vi "_OP_40.vi"(9 "OP_40_Integer":u16[][](array[numeric])=[[0, 0], [0, 0], [0, 0], [0, 0], [0, 0], [0, 0], [0, 0], [0, 0], [0, 0], [0, 0], [0, 0], [0, 0], [0, 0], [0, 0], [0, 0], [52429, 16268], [52429, 16268], [0, 0], [0, 0], [0, 0], [0, 0], [0, 0], [0, 0], [0, 0], [0, 0], [0, 0], [0, 0]], 10 "OP_40_Float":sgl[][](array[numeric])=[[0.0], [0.0], [0.0], [0.0], [1.38], [88.84], [0.0], [11.91], [16.25], [0.0], [0.0], [0.0], [0.0], [-30.7], [30.7], [0.0], [0.0], [-21.4], [26.7], [4.4], [21.91], [6.25], [0.0], [0.0], [0.0], [0.0], [0.0]], 11 "OP_40_string":string[](array[string])) -> (0 "Cluster":T1, 1 "Cluster 2":T1, 2 "Cluster 3":T1, 3 "Cluster 4":T1)   [LabVIEW 2024]
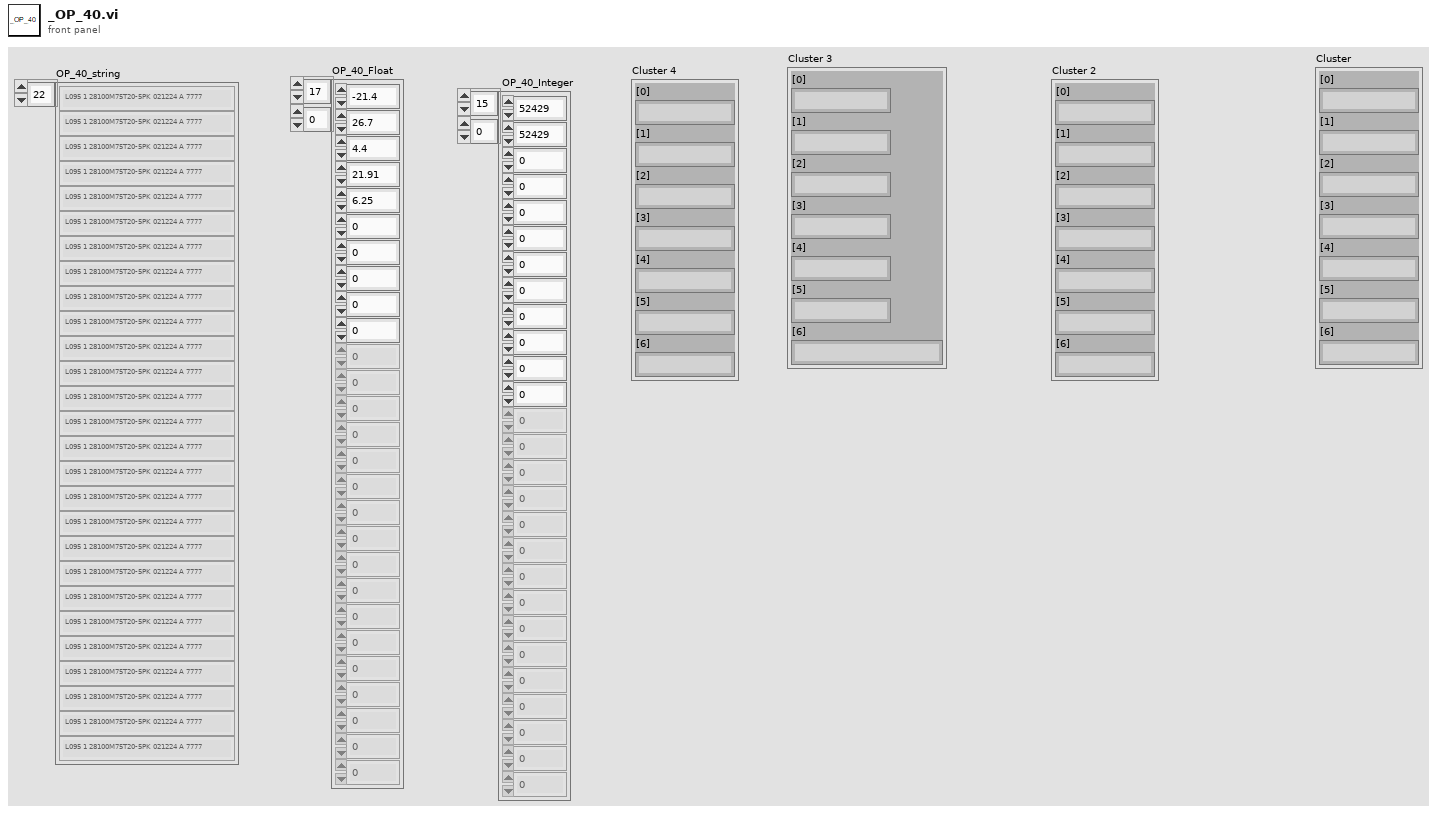
[diagram p1: front panel]
types:
  T1 = cluster{"[0]":string, "[1]":string, "[2]":string, "[3]":string, "[4]":string, "[5]":string, "[6]":string}
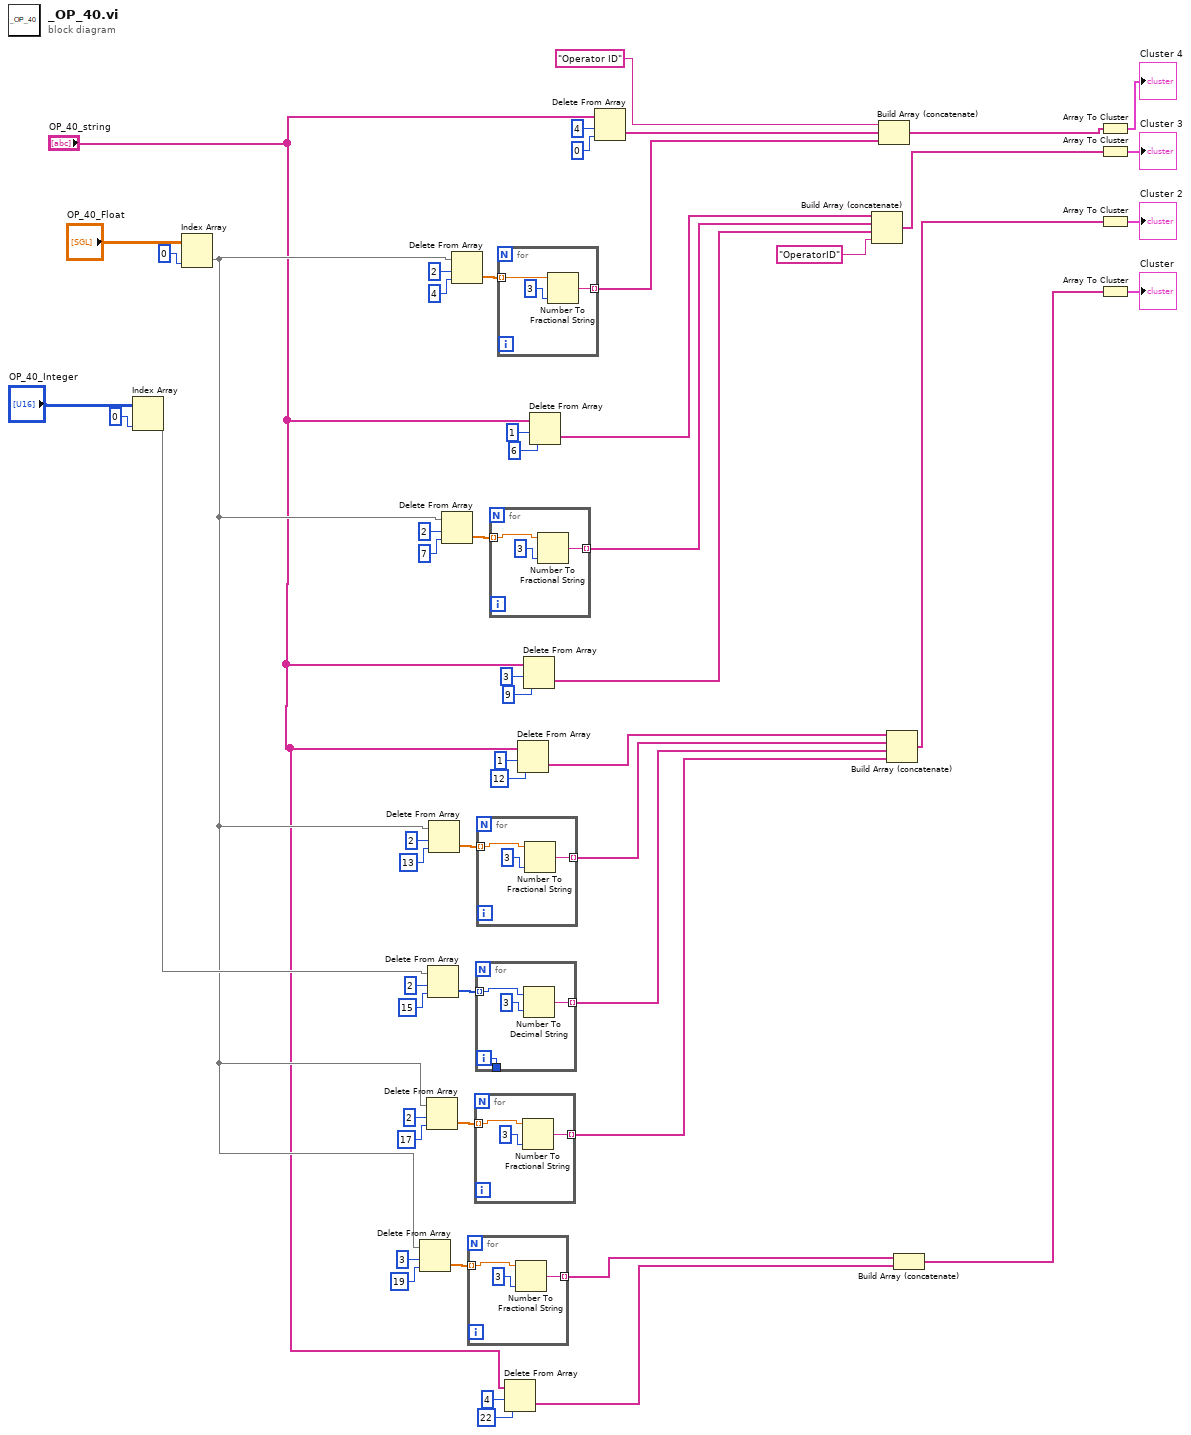
[diagram p0: block diagram]
diagram:
  n1 = Index Array(array="OP_40_Integer", index (col)=0 ("disabled index (col)")) -> (element=w17:u16[])  [unwired: 1 in]
  n2 = Index Array(array="OP_40_Float", index (col)=0 ("disabled index (col)")) -> (element=w7:sgl[])  [unwired: 1 in]
  n3 = Delete From Array(array=w7, length=3, index=19) -> (deleted portion=w10:sgl[])  [unwired: 1 out]
  n4 = Delete From Array(array=w7, length=2, index=17) -> (deleted portion=w13:sgl[])  [unwired: 1 out]
  n5 = Delete From Array(array=w17, length=2, index=15) -> (deleted portion=w20:u16[])  [unwired: 1 out]
  n6 = Delete From Array(array=w7, length=2, index=13) -> (deleted portion=w27:sgl[])  [unwired: 1 out]
  n7 = Delete From Array(array=w7, length=2, index=7) -> (deleted portion=w36:sgl[])  [unwired: 1 out]
  n8 = Delete From Array(array=w7, length=2, index=4) -> (deleted portion=w49:sgl[])  [unwired: 1 out]
  n9 = for {
    tunnel: w10 -> [w57] mode=indexing
    tunnel: [w59] -> w6 mode=indexing
    n10 = Number To Fractional String(number=w57, precision (6)=i16 3) -> (F-format string=w59:string)  [unwired: 2 in]
  }
  n11 = for {
    tunnel: w13 -> [w60] mode=indexing
    tunnel: [w62] -> w12 mode=indexing
    n12 = Number To Fractional String(number=w60, precision (6)=i16 3) -> (F-format string=w62:string)  [unwired: 2 in]
  }
  n13 = for {
    tunnel: w20 -> [w64] mode=indexing
    tunnel: [w66] -> w16 mode=indexing
    tunnel: [w63] -> _
    i -> [w63]
    n14 = Number To Decimal String(number=w64, width (-)=i16 3 ("precision (6)")) -> (decimal integer string=w66:string)
  }
  n15 = for {
    tunnel: w27 -> [w67] mode=indexing
    tunnel: [w69] -> w23 mode=indexing
    n16 = Number To Fractional String(number=w67, precision (6)=i16 3) -> (F-format string=w69:string)  [unwired: 2 in]
  }
  n17 = for {
    tunnel: w36 -> [w70] mode=indexing
    tunnel: [w72] -> w32 mode=indexing
    n18 = Number To Fractional String(number=w70, precision (6)=i16 3) -> (F-format string=w72:string)  [unwired: 2 in]
  }
  n19 = for {
    tunnel: w49 -> [w74] mode=indexing
    tunnel: [w75] -> w51 mode=indexing
    n20 = Number To Fractional String(number=w74, precision (6)=i16 3) -> (F-format string=w75:string)  [unwired: 2 in]
  }
  n21 = Delete From Array(array="OP_40_string", length=4, index=22) -> (deleted portion=w2:string[])  [unwired: 1 out]
  n22 = Delete From Array(array="OP_40_string", length=1, index=12) -> (deleted portion=w24:string[])  [unwired: 1 out]
  n23 = Delete From Array(array="OP_40_string", length=3, index=9) -> (deleted portion=w31:string[])  [unwired: 1 out]
  n24 = Delete From Array(array="OP_40_string", length=1, index=6) -> (deleted portion=w33:string[])  [unwired: 1 out]
  n25 = Delete From Array(array="OP_40_string", length=4, index=0) -> (deleted portion=w42:string[])  [unwired: 1 out]
  n26 = Build Array (concatenate)(w33, w32, w31, "OperatorID") -> (w34:string[])
  n27 = Build Array (concatenate)("Operator ID", w42, w51) -> (w54:string[])
  n28 = Build Array (concatenate)(w24, w23, w16, w12) -> (w11:string[])
  n29 = Build Array (concatenate)(w6, w2) -> (w1:string[])
  n30 = Array To Cluster(array=w54) -> (cluster=→"Cluster 4":T1)
  n31 = Array To Cluster(array=w34) -> (cluster=→"Cluster 3":T1)
  n32 = Array To Cluster(array=w11) -> (cluster=→"Cluster 2":T1)
  n33 = Array To Cluster(array=w1) -> (cluster=→"Cluster":T1)
